vi "Left Click.vi"(7 "object refs":T2, 8 "error in (no error)":errorcluster, 9 "Coords":T1, 10 "Event data":variant, 11 "Table Manager in":refnum<class "Table Manager.lvclass">) -> (0 "error out":errorcluster, 2 "Discard?":bool, 3 "Table Manager out":refnum<class "Table Manager.lvclass">)   [LabVIEW 2013, in "Table Manager.lvlib" / "Table Manager.lvclass"]
uses:
  Table Manager.lvclass
  object ref.ctl
  <vilib>/NI/DCAF/Tag Editor Core/Configuration Editor/Classes/Engine Parent/Engine Parent Editor Node.lvclass
  <vilib>/NI/DCAF/Tag Editor Core/Configuration Editor/Classes/Module editor node/module editor node.lvclass
  <vilib>/Utility/miscctls.llb/LVPoint32TypeDef.ctl
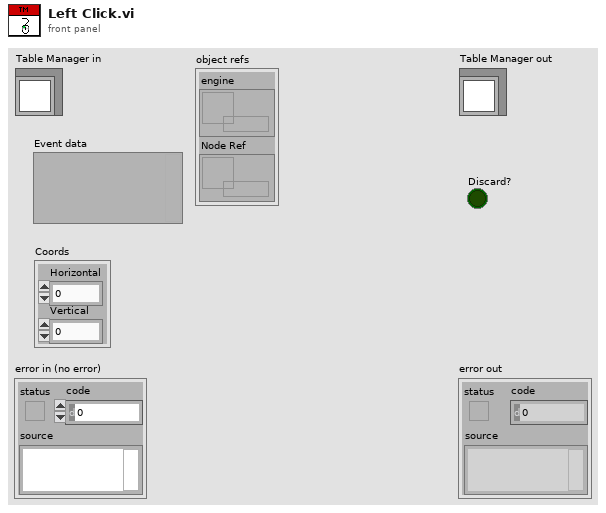
[diagram p1: front panel]
types:
  T1 = typedef "LVPoint32TypeDef.ctl" = cluster{"Horizontal":i32, "Vertical":i32}
  T2 = typedef "Table Manager.lvlib/Table Manager.lvclass/object ref.ctl" = cluster{"engine":refnum<data-value>, "Node Ref":refnum<data-value>}
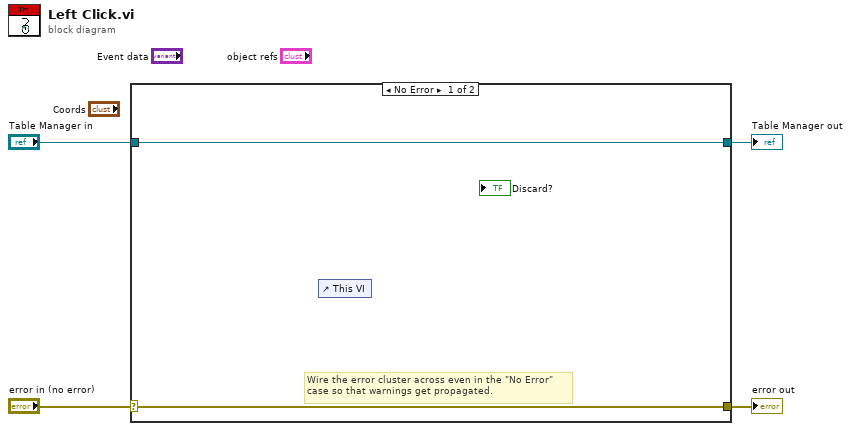
[diagram p0: block diagram]
diagram:
  n1 = case shown="No Error" "error in (no error)" {
    selector: "error in (no error)" -> [w5 w8]
    tunnel: [w5 w8] -> w3
    tunnel: [w6 w7] -> w1
    tunnel: "Table Manager in" -> [w6 w7]
    frame No Error {
      # "Wire the error cluster across even in the \"No Error\"\ncase so that warnings get propagated."
      n2 = control-ref of="This VI"() -> ()  [unwired: 1 out]
    }
    frame Error {
    }
  }
  "error out" <- w3
  "Table Manager out" <- w1
